vi "导出参数设置4.0.vi"(10 "输入":T1) -> ()   [LabVIEW 2016]
uses:
  <vilib>/Utility/config.llb/Write Key (String).vi
  <vilib>/Utility/config.llb/Write Key (Double).vi
  <vilib>/Utility/config.llb/NI_LVConfig.lvlib
panel:
  in  "保存名称":string
  in  "ESC":bool
  in  "OK":bool
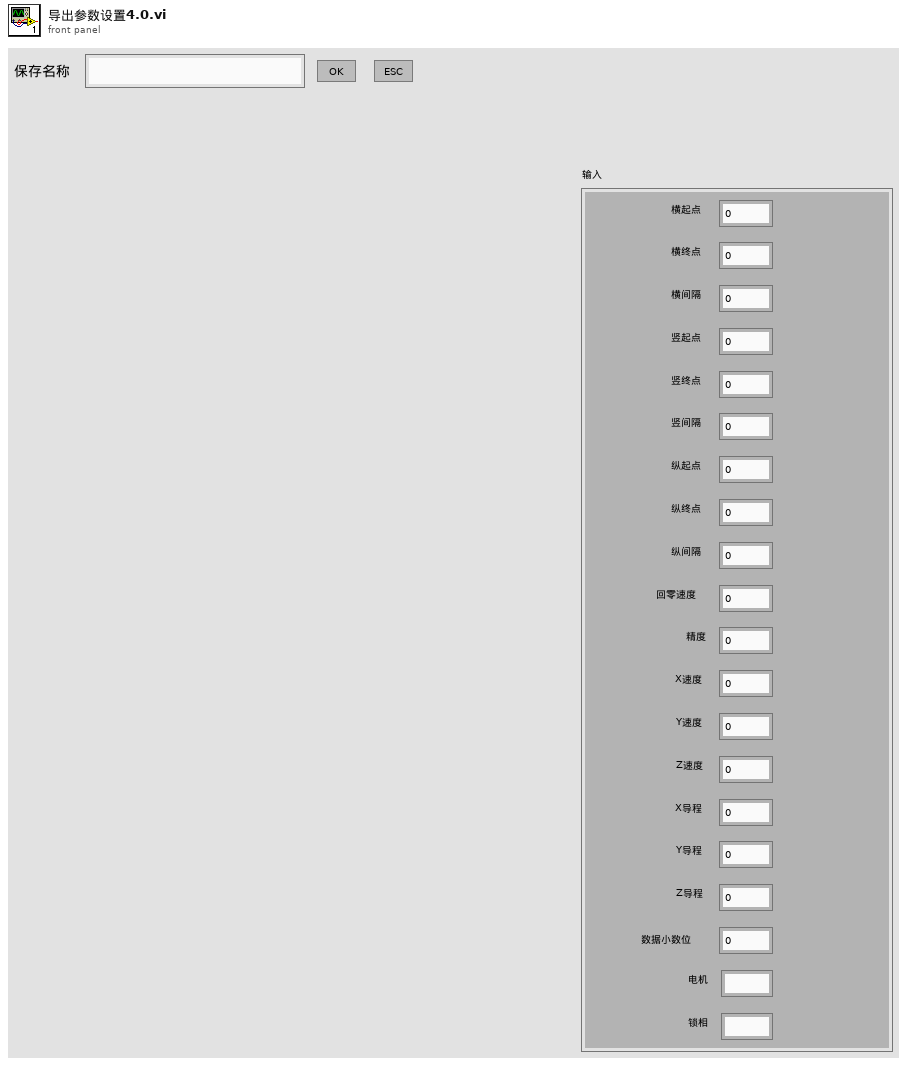
[diagram p1: front panel]
types:
  T1 = cluster{"横起点":dbl, "横终点":dbl, "横间隔":dbl, "竖起点":dbl, "竖终点":dbl, "竖间隔":dbl, "纵起点":dbl, "纵终点":dbl, "纵间隔":dbl, "回零速度":dbl, "精度":dbl, "X速度":dbl, "Y速度":dbl, "Z速度":dbl, "X导程":dbl, "Y导程":dbl, "Z导程":dbl, "数据小数位":dbl, "电机":string, "锁相":string}
  T2 = typedef "NI_LVConfig.lvlib/Config Data RefNum.ctl" = refnum<k1>
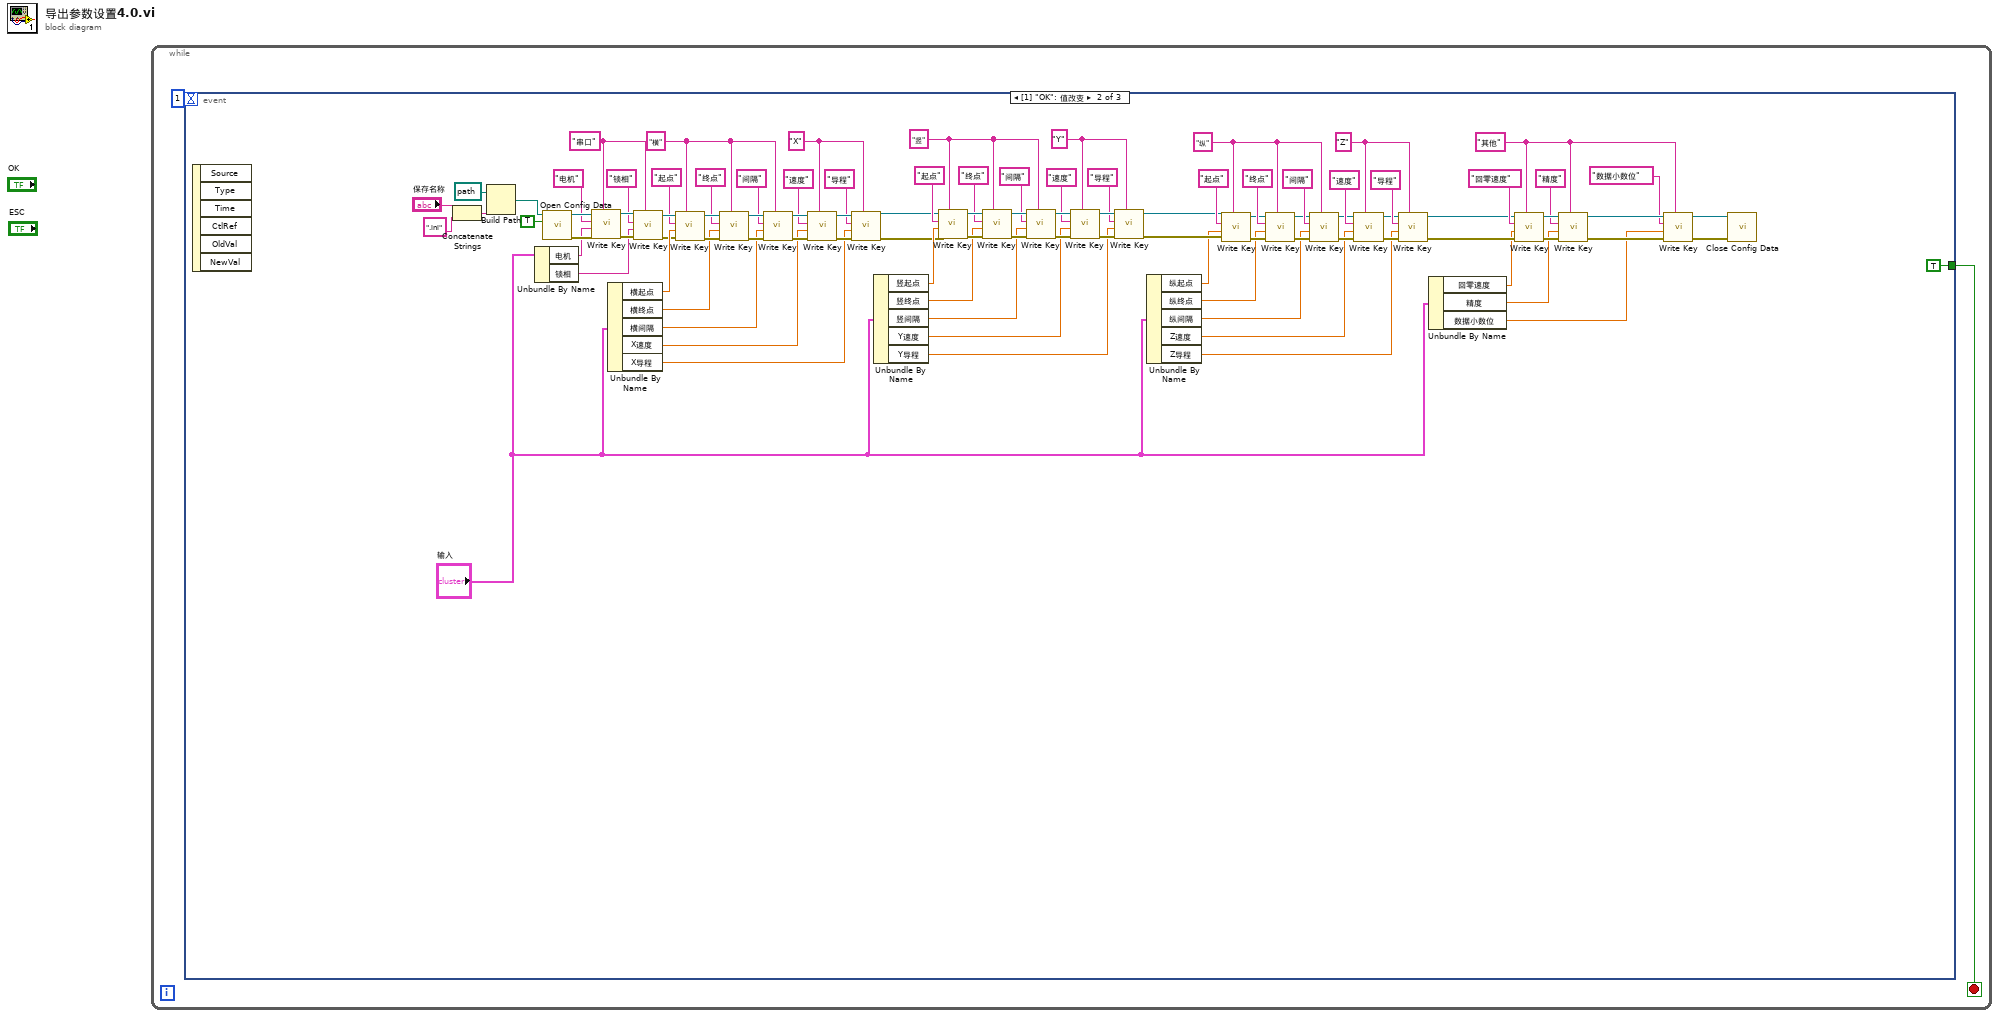
[diagram p0: block diagram]
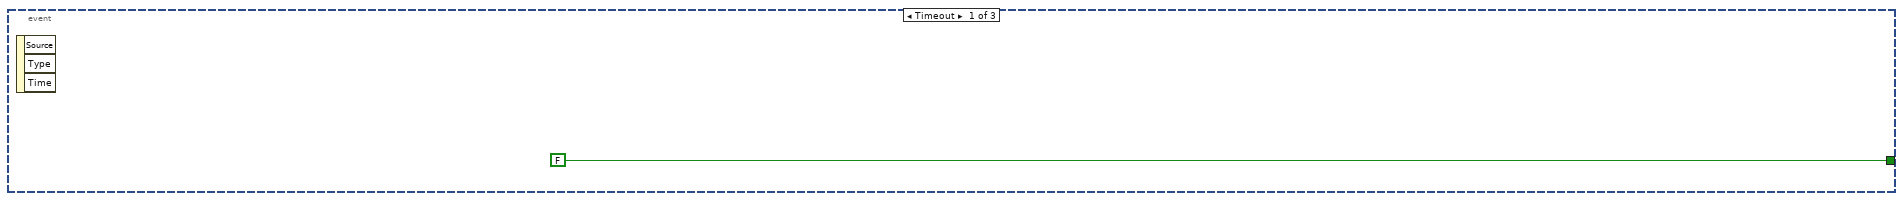
[diagram p2: hidden frame]
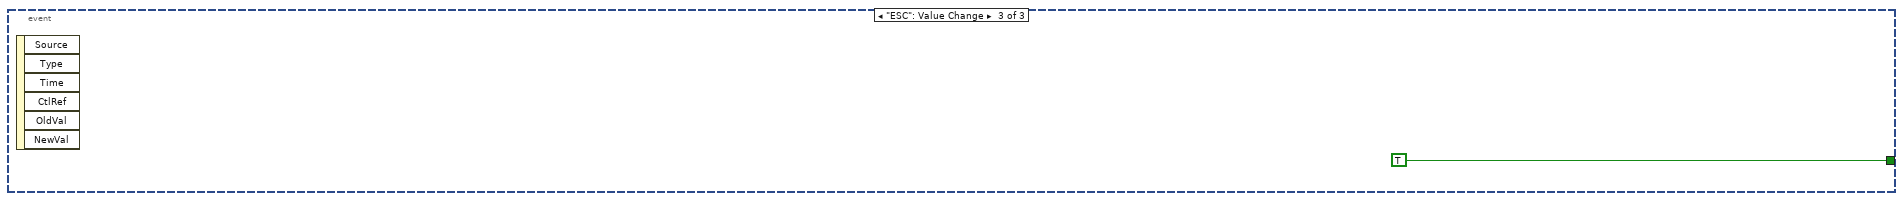
[diagram p3: hidden frame]
diagram:
  n1 = while {
    stop <- w1 stop-if-true
    n2 = event shown="[1] \"OK\": 值改变" {
      selector: _ -> [_ _ _]
      dyn-events: _ -> [_ _ _]
      timeout: 1 -> [_ _ _]
      tunnel: [FALSE TRUE TRUE] -> w1
      event Timeout {
        n3 = event-data() -> ()  [unwired: 1 in, 3 out]
      }
      event "OK": Value Change {
        w20 = "其他" ("section")
        w44 = "Y" ("section")
        w45 = "竖" ("section")
        w63 = "Z" ("section")
        w62 = "纵" ("section")
        w80 = "X" ("section")
        w86 = "横" ("section")
        w97 = "串口" ("section")
        n4 = event-data() -> ()  [unwired: 1 in, 6 out]
        n5 = Concatenate Strings("保存名称", ".ini" ("字符串")) -> (w7:string)
        n6 = Build Path(base path=path "D:/锁相连续采集升级版/配置文件（ini）" ("路径"), name or relative path=w7) -> (appended path=w6:path)
        n7 = Unbundle By Name("输入") -> ("电机"=w84:string, "锁相"=w85:string)
        n8 = call <vilib>:"Open Config Data.vi"("create file if necessary (T)"=TRUE, "configuration file path"=w6) -> ("error out"=w92:errorcluster, "refnum"=w99:T2)  [unwired: 7 in, 1 out]
        n9 = call-poly <vilib>:"Write Key.vi"("section"=w97, "error in (no error)"=w92, "value"=w84, "key"="电机", "refnum"=w99) -> ("error out"=w91:errorcluster, "refnum out"=w98:T2)  [unwired: 4 in, 1 out]
        n10 = Unbundle By Name("输入") -> ("横起点"=w74:dbl, "横终点"=w72:dbl, "横间隔"=w71:dbl, "X速度"=w70:dbl, "X导程"=w69:dbl)
        n11 = call-poly <vilib>:"Write Key.vi"("section"=w97, "error in (no error)"=w91, "value"=w85, "key"="锁相", "refnum"=w98) -> ("error out"=w73:errorcluster, "refnum out"=w81:T2)  [unwired: 4 in, 1 out]
        n12 = call-poly <vilib>:"Write Key.vi"("section"=w86, "error in (no error)"=w73, "value"=w74, "key"="起点", "refnum"=w81) -> ("error out"=w96:errorcluster, "refnum out"=w95:T2)  [unwired: 4 in, 1 out]
        n13 = call-poly <vilib>:"Write Key.vi"("section"=w86, "error in (no error)"=w96, "value"=w72, "key"="终点", "refnum"=w95) -> ("error out"=w94:errorcluster, "refnum out"=w93:T2)  [unwired: 4 in, 1 out]
        n14 = call-poly <vilib>:"Write Key.vi"("section"=w86, "error in (no error)"=w94, "value"=w71, "key"="间隔", "refnum"=w93) -> ("error out"=w88:errorcluster, "refnum out"=w90:T2)  [unwired: 4 in, 1 out]
        n15 = call-poly <vilib>:"Write Key.vi"("section"=w80, "error in (no error)"=w88, "value"=w70, "key"="速度", "refnum"=w90) -> ("error out"=w87:errorcluster, "refnum out"=w89:T2)  [unwired: 4 in, 1 out]
        n16 = call-poly <vilib>:"Write Key.vi"("section"=w80, "error in (no error)"=w87, "value"=w69, "key"="导程", "refnum"=w89) -> ("error out"=w37:errorcluster, "refnum out"=w36:T2)  [unwired: 4 in, 1 out]
        n17 = Unbundle By Name("输入") -> ("竖起点"=w38:dbl, "竖终点"=w35:dbl, "竖间隔"=w34:dbl, "Y速度"=w33:dbl, "Y导程"=w32:dbl)
        n18 = call-poly <vilib>:"Write Key.vi"("section"=w45, "error in (no error)"=w37, "value"=w38, "key"="起点", "refnum"=w36) -> ("error out"=w53:errorcluster, "refnum out"=w52:T2)  [unwired: 4 in, 1 out]
        n19 = call-poly <vilib>:"Write Key.vi"("section"=w45, "error in (no error)"=w53, "value"=w35, "key"="终点", "refnum"=w52) -> ("error out"=w51:errorcluster, "refnum out"=w50:T2)  [unwired: 4 in, 1 out]
        n20 = call-poly <vilib>:"Write Key.vi"("section"=w45, "error in (no error)"=w51, "value"=w34, "key"="间隔", "refnum"=w50) -> ("error out"=w47:errorcluster, "refnum out"=w49:T2)  [unwired: 4 in, 1 out]
        n21 = call-poly <vilib>:"Write Key.vi"("section"=w44, "error in (no error)"=w47, "value"=w33, "key"="速度", "refnum"=w49) -> ("error out"=w46:errorcluster, "refnum out"=w48:T2)  [unwired: 4 in, 1 out]
        n22 = call-poly <vilib>:"Write Key.vi"("section"=w44, "error in (no error)"=w46, "value"=w32, "key"="导程", "refnum"=w48) -> ("error out"=w30:errorcluster, "refnum out"=w31:T2)  [unwired: 4 in, 1 out]
        n23 = Unbundle By Name("输入") -> ("纵起点"=w29:dbl, "纵终点"=w28:dbl, "纵间隔"=w27:dbl, "Z速度"=w26:dbl, "Z导程"=w25:dbl)
        n24 = call-poly <vilib>:"Write Key.vi"("section"=w62, "error in (no error)"=w30, "value"=w29, "key"="起点", "refnum"=w31) -> ("error out"=w54:errorcluster, "refnum out"=w55:T2)  [unwired: 4 in, 1 out]
        n25 = call-poly <vilib>:"Write Key.vi"("section"=w62, "error in (no error)"=w54, "value"=w28, "key"="终点", "refnum"=w55) -> ("error out"=w56:errorcluster, "refnum out"=w57:T2)  [unwired: 4 in, 1 out]
        n26 = call-poly <vilib>:"Write Key.vi"("section"=w62, "error in (no error)"=w56, "value"=w27, "key"="间隔", "refnum"=w57) -> ("error out"=w60:errorcluster, "refnum out"=w58:T2)  [unwired: 4 in, 1 out]
        n27 = call-poly <vilib>:"Write Key.vi"("section"=w63, "error in (no error)"=w60, "value"=w26, "key"="速度", "refnum"=w58) -> ("error out"=w61:errorcluster, "refnum out"=w59:T2)  [unwired: 4 in, 1 out]
        n28 = call-poly <vilib>:"Write Key.vi"("section"=w63, "error in (no error)"=w61, "value"=w25, "key"="导程", "refnum"=w59) -> ("error out"=w15:errorcluster, "refnum out"=w16:T2)  [unwired: 4 in, 1 out]
        n29 = Unbundle By Name("输入") -> ("回零速度"=w14:dbl, "精度"=w13:dbl, "数据小数位"=w12:dbl)
        n30 = call-poly <vilib>:"Write Key.vi"("section"=w20, "error in (no error)"=w15, "value"=w14, "key"="回零速度", "refnum"=w16) -> ("error out"=w24:errorcluster, "refnum out"=w23:T2)  [unwired: 4 in, 1 out]
        n31 = call-poly <vilib>:"Write Key.vi"("section"=w20, "error in (no error)"=w24, "value"=w13, "key"="精度", "refnum"=w23) -> ("error out"=w22:errorcluster, "refnum out"=w21:T2)  [unwired: 4 in, 1 out]
        n32 = call-poly <vilib>:"Write Key.vi"("section"=w20, "error in (no error)"=w22, "value"=w12, "key"="数据小数位", "refnum"=w21) -> ("error out"=w11:errorcluster, "refnum out"=w10:T2)  [unwired: 4 in, 1 out]
        n33 = call <vilib>:"Close Config Data.vi"("error in (no error)"=w11, "refnum"=w10) -> ()  [unwired: 8 in, 2 out]
      }
      event "ESC": Value Change {
        n34 = event-data() -> ()  [unwired: 1 in, 6 out]
      }
    }
  }
